vi "Score L2.vi"(9 "Combo Box":string(combo)) -> (0 "Done":bool)   [LabVIEW 2020]
uses:
  <vilib>/Rock Robotics/WPI/Utilities/WPI_GetSetVariantRefNum.vi
  Robot Global Data.vi
  <vilib>/Rock Robotics/WPI/RobotDrive/WPI_RobotDriveArcadeDrive_Standard(NoSaturation).vi
panel:
  out "Done 2":bool
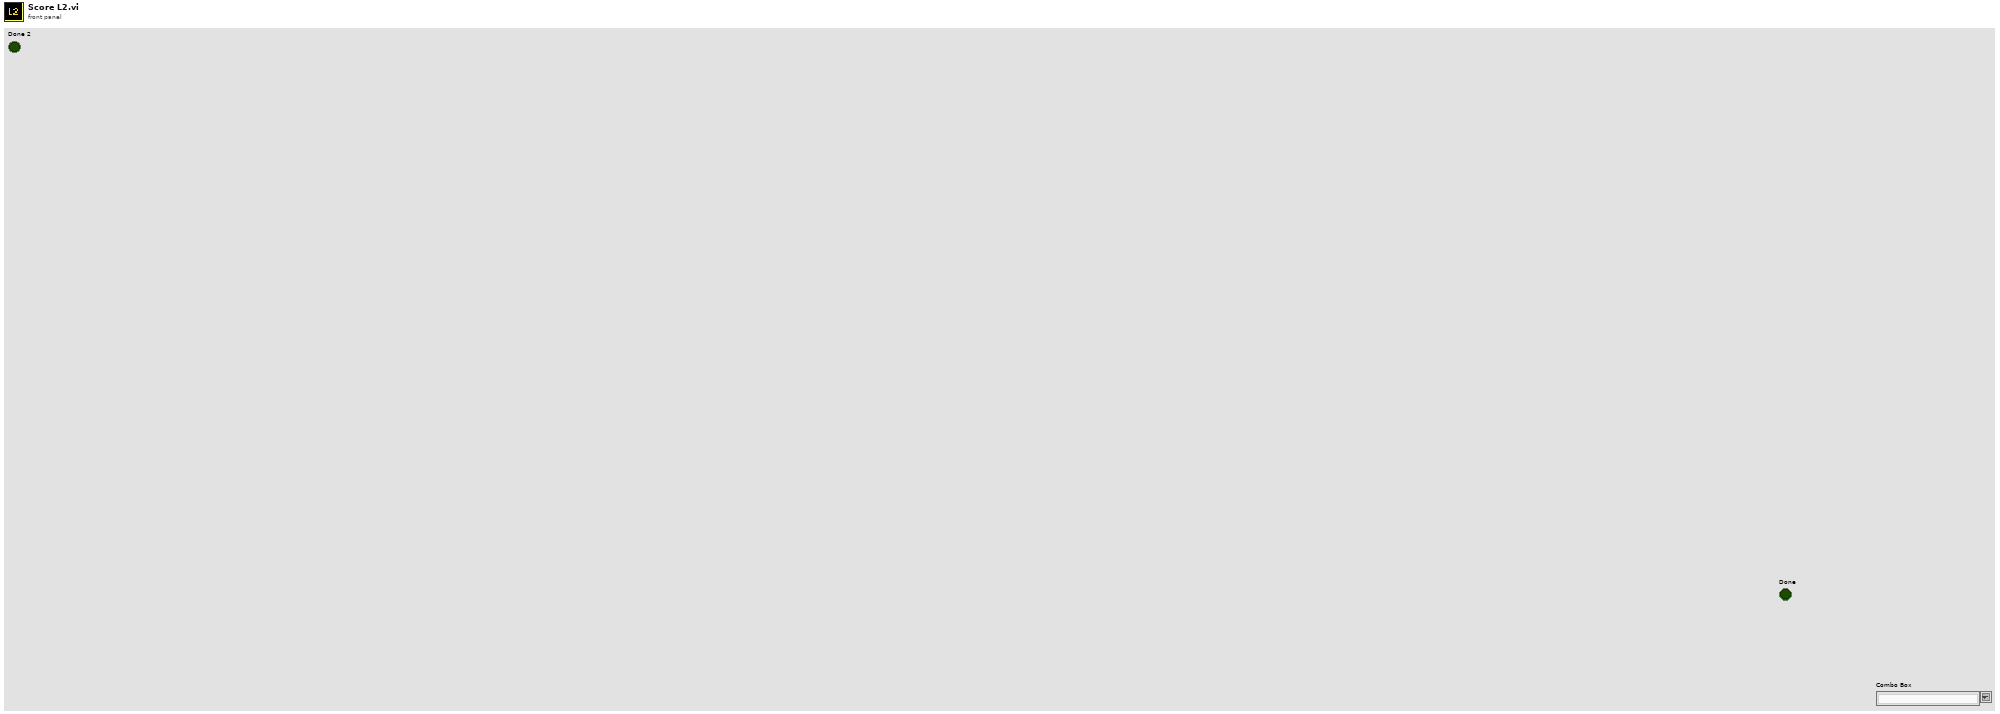
[diagram p1: front panel]
types:
  T1 = typedef "WPI_MotorControlDeviceRef.ctl" = cluster{"DeviceStatus":errorcluster, "Type":T2, "PWM":cluster{"PWM Channel":T3, "DeadBand":T4}, "CAN":cluster{"Device Number":u8, "SetOutput VI Ref":variant, "GetOutput VI Ref":variant, "Enable VI Ref":variant, "Disable VI Ref":variant, "Data":variant}, "Invert":bool, "DIO PWM":cluster{"PWM \"Enable\" Channel":T3, "DIOChannel":T5, "PWM Rate":dbl}}
  T2 = typedef "WPI_MotorControlType.ctl" = enum16{"PWM", "CAN", "DIO PWM"}
  T3 = typedef "FPGA_DIOPWMChannel.ctl" = enum8{"PWM 0", "PWM 1", "PWM 2", "PWM 3", "PWM 4", "PWM 5", "PWM 6", "PWM 7", "PWM 8", "PWM 9", "PWM MXP 0", "PWM MXP 1", "PWM MXP 2", "PWM MXP 3", "PWM MXP 4", "PWM MXP 5", "PWM MXP 6", "PWM MXP 7", "PWM MXP 8", "PWM MXP 9", "Invalid"}
  T4 = typedef "WPI_PWMDeadband.ctl" = cluster{"Name":string, "maxPositivePwm":i32, "minPositivePwm":i32, "centerPwm":i32, "maxNegativePwm":i32, "minNegativePwm":i32, "angularRange":u16}
  T5 = typedef "FPGA_DIOChannel.ctl" = enum8{"DIO 0", "DIO 1", "DIO 2", "DIO 3", "DIO 4", "DIO 5", "DIO 6", "DIO 7", "DIO 8", "DIO 9", "DIO MXP 0", "DIO MXP 1", "DIO MXP 2", "DIO MXP 3", "DIO MXP 4", "DIO MXP 5", "DIO MXP 6", "DIO MXP 7", "DIO MXP 8", "DIO MXP 9", "DIO MXP 10", "DIO MXP 11", "DIO MXP 12", "DIO MXP 13", "DIO MXP 14", "DIO MXP 15", "SPI Port CS1", "SPI Port CS2", "SPI Port CS3", "SPI Port MISO", "SPI Port MOSI", "Invalid"}
  T6 = typedef "ADIS16470 Device Reference.ctl" = cluster{"DevStatus":errorcluster, "Hardware Config":T7, "Calibration Complete":refnum<notifier>, "Status Reference":refnum<data-value>, "Data Reference":refnum<data-value>, "Sychronous Process VI":T10, "Cmd FIFO":refnum<k33>, "Source":T11, "Data FIFO":refnum<k33>, "Calibration Time (ms)":u32, "Data Reference":refnum<data-value>}
  T7 = typedef "ADIS16470 Hardware Configuration.ctl" = cluster{"SPI Clock Rate (Hz)":dbl, "IMU SPI Mode (3)":T8, "IMU Reset Pin":T5, "IMU SPI Bus":T9, "IMU Data Ready Pin":T5, "Stall Config":cluster{"Pow2BytesPerRead":u8, "StallTicks":u16, "CsToSclkTicks":u8}}
  T8 = typedef "WPI_SPIMode.ctl" = enum16{"Mode 0 (Clk Idle Low,Sample on Leading)", "Mode 1 (Clk Idle Low,Sample on Trailing)", "Mode 2 (Clk Idle High,Sample on Leading)", "Mode 3 (Clk Idle High,Sample on Trailing)"}
  T9 = typedef "spi_bus.ctl" = enum16{"SPI On-Board, CS0", "SPI On-Board, CS1", "SPI On-Board, CS2", "SPI On-Board, CS3", "SPI MXP", "Invalid"}
  T10 = typedef "ADIS16470 Process.ctl" = refnum<vi>
  T11 = typedef "FPGA_CounterEncoderSourceConvertionLVSourceType.ctl" = cluster{"DevStatus":errorcluster, "AnalogTriggerMode?":bool, "DigitalMode":cluster{"DIO Channel":T12}, "AnalogTriggerMode":cluster{"AnalogTriggerIndex":T13, "OutputType":T14}}
  T12 = typedef "FPGA_DIODigitalSourceChannel.ctl" = enum8{"DIO 0", "DIO 1", "DIO 2", "DIO 3", "DIO 4", "DIO 5", "DIO 6", "DIO 7", "DIO 8", "DIO 9", "DIO MXP 0", "DIO MXP 1", "DIO MXP 2", "DIO MXP 3", "DIO MXP 4", "DIO MXP 5", "DIO MXP 6", "DIO MXP 7", "DIO MXP 8", "DIO MXP 9", "DIO MXP 10", "DIO MXP 11", "DIO MXP 12", "DIO MXP 13", "DIO MXP 14", "DIO MXP 15", "SPI Port CS1", "SPI Port CS2", "SPI Port CS3", "SPI Port MISO", "SPI Port MOSI", "Disabled"}
  T13 = typedef "FPGA_AnalogTriggerIndex.ctl" = enum8{"Trig 0", "Trig 1", "Trig 2", "Trig 3", "Trig 4", "Trig 5", "Trig 6", "Trig 7", "Invalid"}
  T14 = typedef "FPGA_AnalogTriggerOutType.ctl" = enum16{"InWindow", "TriggerState", "Rising", "Falling"}
  T15 = typedef "WPI_RobotDriveDevRef.ctl" = cluster{"DevStatus":errorcluster, "Motors[]":T1[], "Square Inputs":bool, "Max Output":dbl}
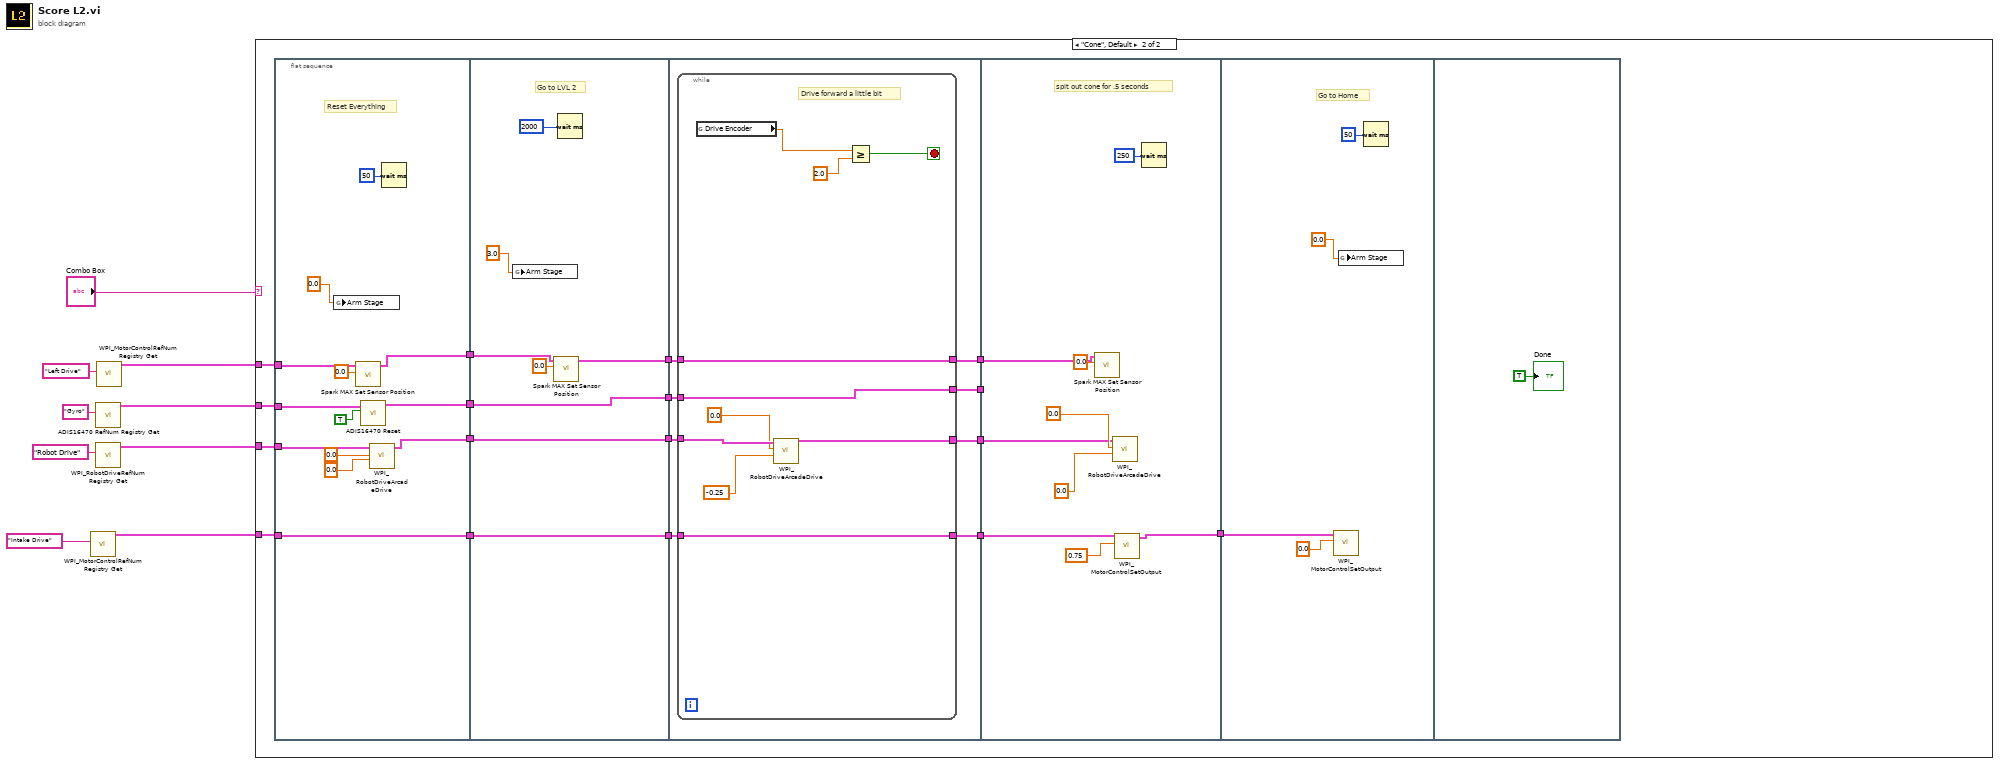
[diagram p0: block diagram]
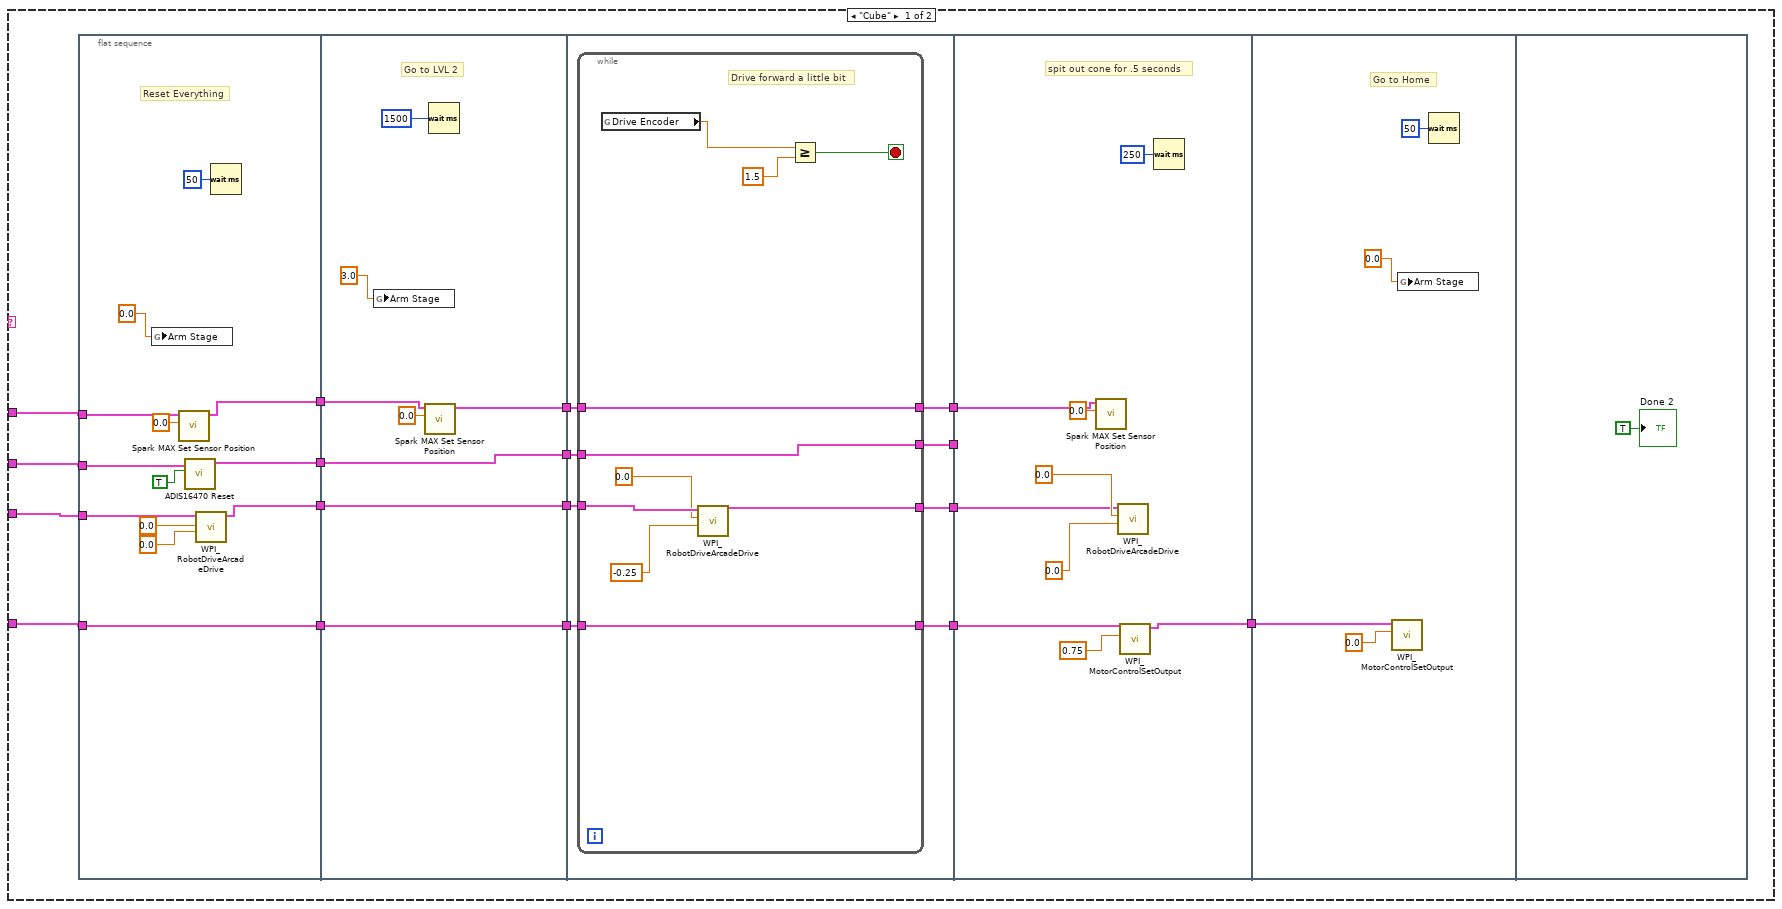
[diagram p2: hidden frame]
diagram:
  n1 = call <vilib>:"WPI_MotorControlRefNum Registry Get.vi"("refnum name"="Intake Drive") -> ("MotorControlDevRef"=w2:T1)  [unwired: 9 in, 1 out]
  n2 = call <vilib>:"ADIS16470 RefNum Registry Get.vi"("refnum name"="Gyro") -> ("ADIS16470DevRef out"=w4:T6)  [unwired: 9 in, 1 out]
  n3 = call <vilib>:"WPI_RobotDriveRefNum Registry Get.vi"("refnum name"="Robot Drive") -> ("RobotDriveDevRef"=w3:T15)  [unwired: 9 in, 1 out]
  n4 = call <vilib>:"WPI_MotorControlRefNum Registry Get.vi"("refnum name"="Left Drive") -> ("MotorControlDevRef"=w5:T1)  [unwired: 9 in, 1 out]
  n5 = case shown="\"Cone\", Default" "Combo Box" {
    tunnel: w5 -> [w10 w90]
    tunnel: w4 -> [w11 w89]
    tunnel: w3 -> [w12 w88]
    tunnel: w2 -> [w13 w87]
    frame "Cube" {
      n6 = flat-sequence {
        tunnel: w12 -> [w39]
        tunnel: w10 -> [w36]
        tunnel: w11 -> [w34]
        tunnel: [w30] -> w26
        tunnel: w13 -> [w27]
        tunnel: [w29] -> w25
        tunnel: [w28] -> w24
        tunnel: [w27] -> w23
        tunnel: [w45] -> w22
        tunnel: w26 -> [w45]
        tunnel: w25 -> [w43]
        tunnel: [w42] -> w21
        tunnel: [w41] -> w20
        tunnel: w24 -> [w41]
        tunnel: w23 -> [w40]
        tunnel: [w40] -> w19
        tunnel: w22 -> [w55]
        tunnel: [w54] -> w18
        tunnel: [w53] -> w17
        tunnel: w21 -> [w52]
        tunnel: [w51] -> w16
        tunnel: w20 -> [w50]
        tunnel: w19 -> [w49]
        tunnel: [w48] -> w15
        tunnel: w18 -> [w71]
        tunnel: w17 -> [w68]
        tunnel: w16 -> [_]
        tunnel: [w67] -> w14
        tunnel: w15 -> [w66]
        tunnel: w14 -> [w76]
        frame #0 {
          # "Reset Everything"
          n7 = global write "Robot Global Data.vi" "Arm Stage"(0.0 ("Arm Stage")) -> ()
          n8 = call <vilib>:"Spark MAX Set Sensor Position.vi"("Position"=0.0, "MotorControlDeviceRef"=w36) -> ("MotorControlDeviceRef"=w29:T1)  [unwired: 8 in, 1 out]
          n9 = call <vilib>:"ADIS16470 Reset.vi"("Reset? (T)"=TRUE, "ADIS16470DevRef"=w34) -> ("ADIS16470DevRef"=w28:T6)  [unwired: 8 in, 1 out]
          n10 = call-poly <vilib>:"WPI_RobotDriveArcadeDrive.vi"("Y axis value"=0.0, "X axis value"=0.0, "RobotDriveDevRef"=w39) -> ("RobotDriveDevRef"=w30:T15)  [unwired: 6 in, 2 out]
          n11 = Wait (ms)(milliseconds to wait=u32 50) -> ()  [unwired: 1 out]
        }
        frame #1 {
          # "Go to LVL 2"
          n12 = global write "Robot Global Data.vi" "Arm Stage"(3.0 ("Arm Stage")) -> ()
          n13 = call <vilib>:"Spark MAX Set Sensor Position.vi"("Position"=0.0, "MotorControlDeviceRef"=w43) -> ("MotorControlDeviceRef"=w42:T1)  [unwired: 8 in, 1 out]
          n14 = Wait (ms)(milliseconds to wait=u32 1500) -> ()  [unwired: 1 out]
        }
        frame #2 {
          n15 = while {
            tunnel: w55 -> [w65]
            tunnel: [w59] -> w54
            tunnel: [w58] -> w53
            tunnel: w52 -> [w58]
            tunnel: [w57] -> w51
            tunnel: w50 -> [w57]
            tunnel: w49 -> [w56]
            tunnel: [w56] -> w48
            stop <- w60 stop-if-true
            # "Drive forward a little bit"
            n16 = global read "Robot Global Data.vi" "Drive Encoder"() -> (w62:dbl)
            n17 = call-poly <vilib>:"WPI_RobotDriveArcadeDrive.vi"("Y axis value"=-0.25, "X axis value"=0.0, "RobotDriveDevRef"=w65) -> ("RobotDriveDevRef"=w59:T15)  [unwired: 6 in, 2 out]
            n18 = Greater Or Equal?(x=w62, y=1.5) -> (x >= y?=w60:bool)
          }
        }
        frame #3 {
          # "spit out cone for .5 seconds"
          n19 = call <vilib>:"Spark MAX Set Sensor Position.vi"("Position"=0.0, "MotorControlDeviceRef"=w68) -> ()  [unwired: 8 in, 2 out]
          n20 = call-poly <vilib>:"WPI_RobotDriveArcadeDrive.vi"("Y axis value"=0.0, "X axis value"=0.0, "RobotDriveDevRef"=w71) -> ()  [unwired: 6 in, 3 out]
          n21 = call <vilib>:"WPI_MotorControlSetOutput.vi"("Output"=0.75, "MotorControlDevRef"=w66) -> ("MotorControlDevRef"=w67:T1)  [unwired: 7 in, 2 out]
          n22 = Wait (ms)(milliseconds to wait=u32 250) -> ()  [unwired: 1 out]
        }
        frame #4 {
          # "Go to Home"
          n23 = call <vilib>:"WPI_MotorControlSetOutput.vi"("Output"=0.0, "MotorControlDevRef"=w76) -> ()  [unwired: 7 in, 3 out]
          n24 = global write "Robot Global Data.vi" "Arm Stage"(0.0 ("Arm Stage")) -> ()
          n25 = Wait (ms)(milliseconds to wait=u32 50) -> ()  [unwired: 1 out]
        }
        frame #5 {
          "Done 2" <- TRUE ("Done")
        }
      }
    }
    frame "Cone", Default {
      n26 = flat-sequence {
        tunnel: w88 -> [w109]
        tunnel: w90 -> [w106]
        tunnel: w89 -> [w104]
        tunnel: [w100] -> w86
        tunnel: w87 -> [w97]
        tunnel: [w99] -> w85
        tunnel: [w98] -> w84
        tunnel: [w97] -> w83
        tunnel: [w115] -> w96
        tunnel: w86 -> [w115]
        tunnel: w85 -> [w113]
        tunnel: [w112] -> w95
        tunnel: [w111] -> w94
        tunnel: w84 -> [w111]
        tunnel: w83 -> [w110]
        tunnel: [w110] -> w82
        tunnel: w96 -> [w125]
        tunnel: [w124] -> w93
        tunnel: [w123] -> w92
        tunnel: w95 -> [w122]
        tunnel: [w121] -> w91
        tunnel: w94 -> [w120]
        tunnel: w82 -> [w119]
        tunnel: [w118] -> w81
        tunnel: w93 -> [w141]
        tunnel: w92 -> [w138]
        tunnel: w91 -> [_]
        tunnel: [w137] -> w80
        tunnel: w81 -> [w136]
        tunnel: w80 -> [w146]
        frame #0 {
          # "Reset Everything"
          n27 = global write "Robot Global Data.vi" "Arm Stage"(0.0 ("Arm Stage")) -> ()
          n28 = call <vilib>:"Spark MAX Set Sensor Position.vi"("Position"=0.0, "MotorControlDeviceRef"=w106) -> ("MotorControlDeviceRef"=w99:T1)  [unwired: 8 in, 1 out]
          n29 = call <vilib>:"ADIS16470 Reset.vi"("Reset? (T)"=TRUE, "ADIS16470DevRef"=w104) -> ("ADIS16470DevRef"=w98:T6)  [unwired: 8 in, 1 out]
          n30 = call-poly <vilib>:"WPI_RobotDriveArcadeDrive.vi"("Y axis value"=0.0, "X axis value"=0.0, "RobotDriveDevRef"=w109) -> ("RobotDriveDevRef"=w100:T15)  [unwired: 6 in, 2 out]
          n31 = Wait (ms)(milliseconds to wait=u32 50) -> ()  [unwired: 1 out]
        }
        frame #1 {
          # "Go to LVL 2"
          n32 = global write "Robot Global Data.vi" "Arm Stage"(3.0 ("Arm Stage")) -> ()
          n33 = call <vilib>:"Spark MAX Set Sensor Position.vi"("Position"=0.0, "MotorControlDeviceRef"=w113) -> ("MotorControlDeviceRef"=w112:T1)  [unwired: 8 in, 1 out]
          n34 = Wait (ms)(milliseconds to wait=u32 2000) -> ()  [unwired: 1 out]
        }
        frame #2 {
          n35 = while {
            tunnel: w125 -> [w135]
            tunnel: [w129] -> w124
            tunnel: [w128] -> w123
            tunnel: w122 -> [w128]
            tunnel: [w127] -> w121
            tunnel: w120 -> [w127]
            tunnel: w119 -> [w126]
            tunnel: [w126] -> w118
            stop <- w130 stop-if-true
            # "Drive forward a little bit"
            n36 = global read "Robot Global Data.vi" "Drive Encoder"() -> (w132:dbl)
            n37 = call-poly <vilib>:"WPI_RobotDriveArcadeDrive.vi"("Y axis value"=-0.25, "X axis value"=0.0, "RobotDriveDevRef"=w135) -> ("RobotDriveDevRef"=w129:T15)  [unwired: 6 in, 2 out]
            n38 = Greater Or Equal?(x=w132, y=2.0) -> (x >= y?=w130:bool)
          }
        }
        frame #3 {
          # "spit out cone for .5 seconds"
          n39 = call <vilib>:"Spark MAX Set Sensor Position.vi"("Position"=0.0, "MotorControlDeviceRef"=w138) -> ()  [unwired: 8 in, 2 out]
          n40 = call-poly <vilib>:"WPI_RobotDriveArcadeDrive.vi"("Y axis value"=0.0, "X axis value"=0.0, "RobotDriveDevRef"=w141) -> ()  [unwired: 6 in, 3 out]
          n41 = call <vilib>:"WPI_MotorControlSetOutput.vi"("Output"=0.75, "MotorControlDevRef"=w136) -> ("MotorControlDevRef"=w137:T1)  [unwired: 7 in, 2 out]
          n42 = Wait (ms)(milliseconds to wait=u32 250) -> ()  [unwired: 1 out]
        }
        frame #4 {
          # "Go to Home"
          n43 = call <vilib>:"WPI_MotorControlSetOutput.vi"("Output"=0.0, "MotorControlDevRef"=w146) -> ()  [unwired: 7 in, 3 out]
          n44 = global write "Robot Global Data.vi" "Arm Stage"(0.0 ("Arm Stage")) -> ()
          n45 = Wait (ms)(milliseconds to wait=u32 50) -> ()  [unwired: 1 out]
        }
        frame #5 {
          "Done" <- TRUE ("Done")
        }
      }
    }
  }
